vi "CAN Get Error Text.vi"(9 "Buffer":string, 10 "Language":u16, 11 "Error":u32) -> (1 "Buffer out":string, 3 "function return":u32)   [LabVIEW 2020, in "PCANBasic.lvlib"]
doc: "TPCANStatus __stdcall CAN_GetErrorText(\n TPCANStatus Error, \n WORD Language, \n LPSTR Buffer);"
uses:
  PCANBasic.lvlib
  <userlib>/PCANBasic/PCANBasic.dll
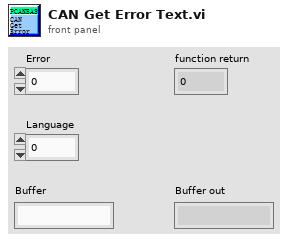
[diagram p1: front panel]
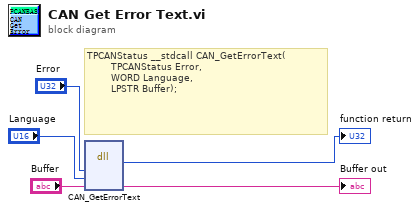
[diagram p0: block diagram]
diagram:
  # "TPCANStatus __stdcall CAN_GetErrorText(\n        TPCANStatus Error, \n        WORD Language, \n        LPSTR Buffer);"
  n1 = dll-call lib="D:/Program Files (x86)/National Instruments/LabVIEW 2020/user.lib/PCANBasic/PCANBasic.*" fn="CAN_GetErrorText"("Error"="Error", "Language"="Language", "Buffer"="Buffer") -> (→"function return":u32, "Buffer"=→"Buffer out":string)  [unwired: 5 in, 2 out]
